vi "FibonacciSeries.vi"() -> ()   [LabVIEW 2020]
panel:
  out "Answer 2":dbl[](array[numeric])
  in  "Limit 2":i32
  out "Answer":dbl[](array[numeric])
  in  "Limit":i32
  # "OUTPUT USING SHIFT REGISTERS"
  # "OUTPUT USING FEEDBACK"
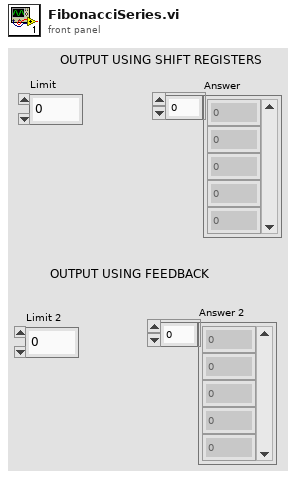
[diagram p1: front panel]
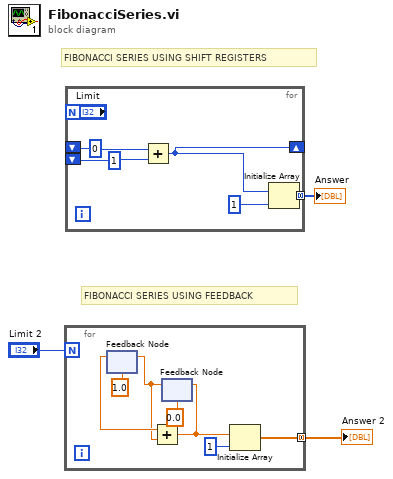
[diagram p0: block diagram]
diagram:
  # "FIBONACCI SERIES USING FEEDBACK"
  # "FIBONACCI SERIES USING SHIFT REGISTERS"
  n1 = for {
    N: "Limit 2" -> [_]
    tunnel: [w13] -> w1 mode=concatenating
    n2 = feedback #1(1.0) -> (w9:dbl)
    n3 = feedback #2(0.0) -> (w7:dbl)
    n4 = feedback-in #1(w7) -> ()
    n5 = Add(x=w9, y=w7) -> (x+y=w10:dbl)
    n6 = feedback-in #2(w10) -> ()
    n7 = Initialize Array(w10, 1 ("dimension size")) -> (w13:dbl[])
  }
  "Answer 2" <- w1
  n8 = for {
    N: "Limit" -> [_]
    shift-right: [w15] -> _
    shift-left: 0 ("Limit 2") -> [w18]
    shift-left: 1 ("Limit 2") -> [w17]
    tunnel: [w16] -> w3 mode=concatenating
    n9 = Add(x=w18, y=w17) -> (x+y=w15:i32)
    n10 = Initialize Array(w15, 1 ("dimension size")) -> (w16:i32[])
  }
  "Answer" <- w3
